vi "TCPGetMulliganList.vi"(1 "error in (no error)":errorcluster, 4 "connection ID":refnum<k5>) -> ()   [LabVIEW 2013]
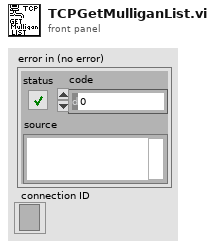
[diagram p1: front panel]
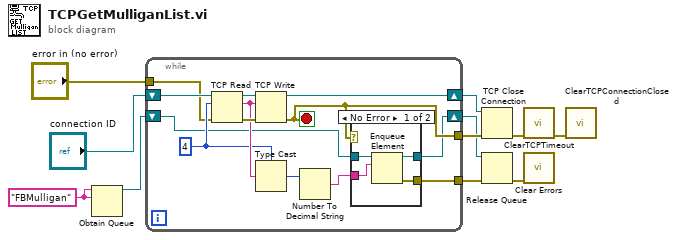
[diagram p0: block diagram]
diagram:
  w7 = "FBMulligan" ("name (unnamed)")
  n1 = Obtain Queue(name (unnamed)=w7, element data type=w7) -> (queue out=w6:refnum<queue>)  [unwired: 3 in, 2 out]
  n2 = while {
    tunnel: [w16] -> w11
    shift-right: [w22] -> w10
    shift-left: "connection ID" -> [w19]
    tunnel: "error in (no error)" -> [w17]
    shift-right: [w13] -> w5
    shift-left: w6 -> [w15]
    tunnel: [w12] -> w4
    stop <- w16 stop-if-true
    w18 = 4
    n3 = TCP Read(connection ID=w19, bytes to read=w18, error in (no error)=w17) -> (connection ID out=w23:refnum<k5>, data out=w21:string, error out=w24:errorcluster)  [unwired: 2 in]
    n4 = TCP Write(connection ID=w23, data in=w21, error in (no error)=w24) -> (connection ID out=w22:refnum<k5>, error out=w16:errorcluster)  [unwired: 1 in, 1 out]
    n5 = Type Cast(type=w18, x=w21) -> (*(type *) &x=w20:i32)
    n6 = Number To Decimal String(number=w20) -> (decimal integer string=w14:string)  [unwired: 1 in]
    n7 = case shown="No Error" w16 {
      tunnel: w15 -> [w27 w29]
      tunnel: w14 -> [w28 _]
      tunnel: [w26 w29] -> w13
      tunnel: [w25 _] -> w12
      frame No Error {
        n8 = Enqueue Element(queue=w27, element=w28) -> (queue out=w26:refnum<queue>, error out=w25:errorcluster)  [unwired: 2 in, 1 out]
      }
      frame Error {
      }
    }
  }
  n9 = TCP Close Connection(connection ID=w10, error in (no error)=w11) -> (error out=w1:errorcluster)  [unwired: 1 in, 1 out]
  n10 = Release Queue(queue=w5, error in (no error)=w4) -> (error out=w3:errorcluster)  [unwired: 1 in, 2 out]
  n11 = call "ClearTCPTimeout.vi"("error in (no error)"=w1) -> ("error out"=w2:errorcluster)  [unwired: 9 in, 1 out]
  n12 = call <vilib>:"Clear Errors.vi"("error in (no error)"=w3) -> ()  [unwired: 6 in, 1 out]
  n13 = call "ClearTCPConnectionClosed.vi"("error in (no error)"=w2) -> ()  [unwired: 9 in, 2 out]
